vi "Remove Color Transform Matrix.vi"(8 "error in (no error)":errorcluster, 10 "index":i32, 11 "ColorProcessor reference in":refnum<k24>) -> (0 "error out":errorcluster, 3 "ColorProcessor reference out":refnum<k24>)   [LabVIEW 2015]
uses:
  C:/code/ScientificCameraInterfaces/Installer/Scientific Camera Interfaces/LabVIEW/64_bit/Library_X64/Thorlabs.TSI.ColorInterfaces.dll
  code/ScientificCameraInterfaces/Installer/Scientific Camera Interfaces/LabVIEW/64_bit/Library_X64/Thorlabs.TSI.ColorInterfaces.dll
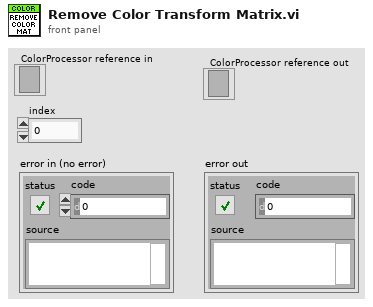
[diagram p1: front panel]
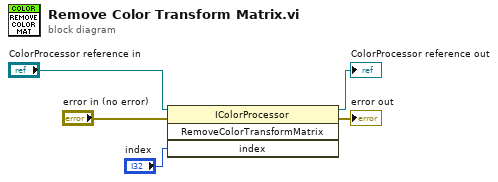
[diagram p0: block diagram]
diagram:
  n1 = invoke class="IColorProcessor" method="RemoveColorTransformMatrix"(reference="ColorProcessor reference in", error in="error in (no error)", "index"="index") -> (reference out=→"ColorProcessor reference out":refnum<k24>, error out=→"error out":errorcluster)  [unwired: 1 in, 2 out]
